vi "SCTL Sector Accumulation.vi"() -> (2 "Accummulated":T1(array[cluster]), 3 "New Data?":bool)   [LabVIEW 2013]
uses:
  Accumulated Count Array Fixed Point.ctl
  <vilib>/rvi/Memory/Memory_Emulation/niFpgaMemoryEmulationReadFromVariant.vi
  <vilib>/rvi/Emulation/niFpgaSctlEmulationGetInTimedLoop.vi
  <vilib>/rvi/Memory/Memory_Emulation/niFpgaMemoryEmulationWriteToVariant.vi
  <vilib>/rvi/DataTransferAndStorage/Container/Common/niFpgaContainerGetUniqueNameForEmu.vi
  <vilib>/rvi/FIFO/Fifo_Resource/nirvififoEmulationSetSize.vi
  <vilib>/rvi/Emulation/niFpgaSctlEmulationFifoFullMgr.vi
  <vilib>/rvi/errors/niFpgaSetErrorForExecOnDevCompSimple.vi
  <vilib>/rvi/eio/common/nirviEmuReportErrorAndStop.vi
  <vilib>/rvi/Emulation/niFpgaSctlEmulationResourceMgr.vi
  <vilib>/rvi/Memory/Memory_Emulation/nirvimemoryFastEmulation.vi
  <vilib>/rvi/Memory/Memory_Emulation/nirvimemoryEmulation.vi
  <vilib>/rvi/DataTransferAndStorage/Container/XNode/niFpgaContainer.xnode
  <vilib>/rvi/FIFO/Fifo_Resource/nirvififoEmulationRead.vi
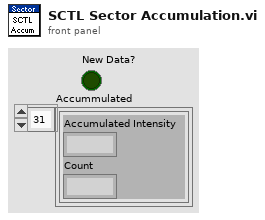
[diagram p1: front panel]
types:
  T1 = cluster{"Accumulated Intensity":fxp<+,20,20>, "Count":fxp<+,12,12>}[]
  T2 = cluster{"Accumulated Intensity":fxp<+,8,8>, "Count":fxp<+,1,1>}
  T3 = typedef "Accumulated Count Array Fixed Point.ctl" = cluster{"Accumulated Intensity":fxp<+,20,20>, "Count":fxp<+,12,12>}[]
  T4 = cluster{"Accumulated Intensity":fxp<+,21,21>, "Count":fxp<+,13,13>}[]
  T5 = cluster{"Accumulated Intensity":fxp<+,22,22>, "Count":fxp<+,14,14>}[]
  T6 = cluster{"Accumulated Intensity":fxp<+,23,23>, "Count":fxp<+,15,15>}[]
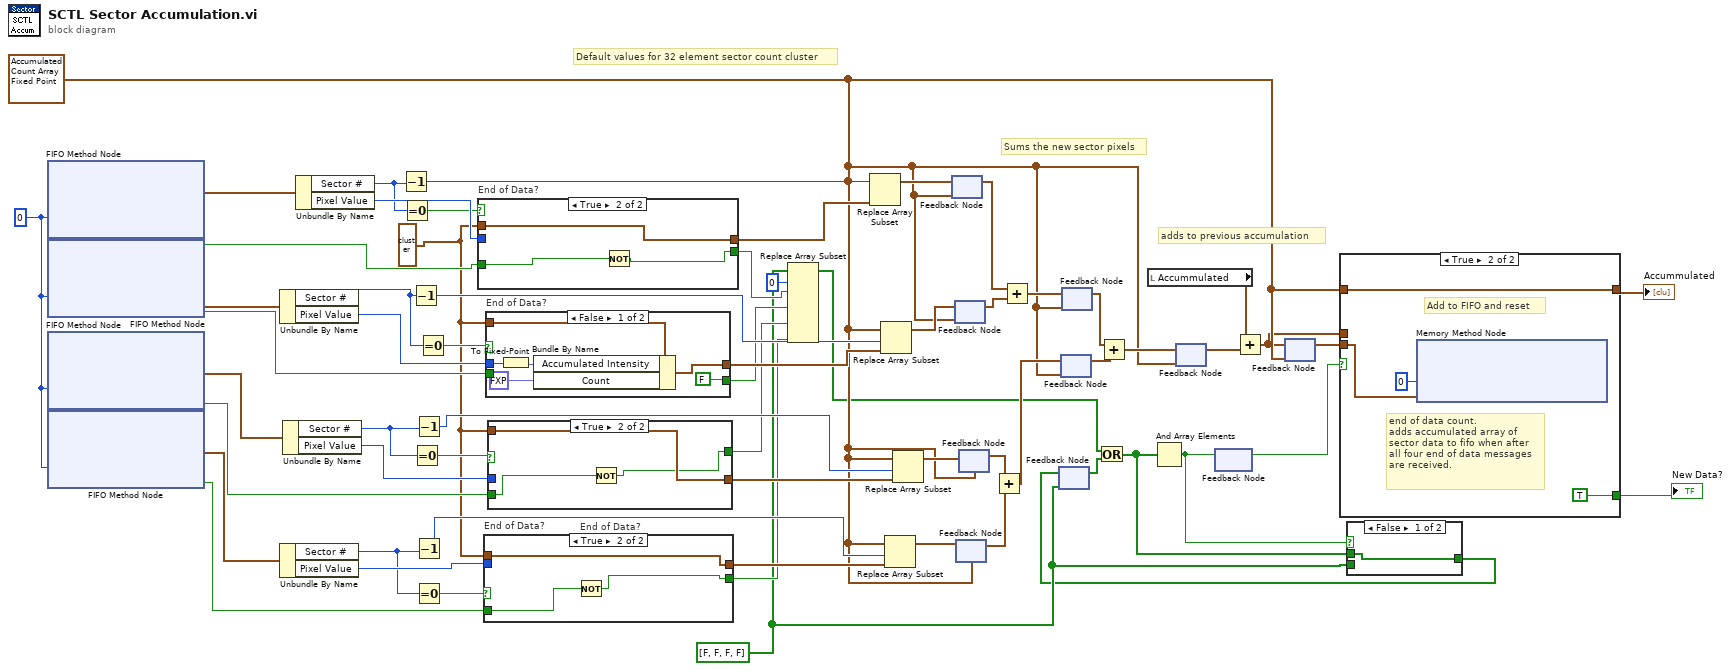
[diagram p0: block diagram]
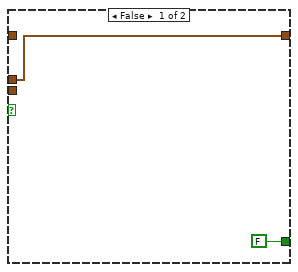
[diagram p3: hidden frame]
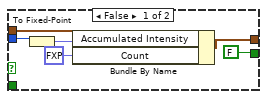
[diagram p4: hidden frame]
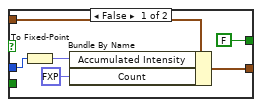
[diagram p5: hidden frame]
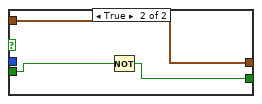
[diagram p6: hidden frame]
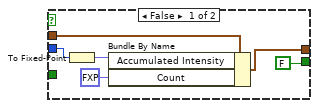
[diagram p7: hidden frame]
diagram:
  w2 = bool[] [FALSE, FALSE, FALSE, FALSE]
  w32 = T2 {"Accumulated Intensity"=0.0, "Count"=0.0} ("Accumulated Sector Cluster")
  w14 = T3 [{"Accumulated Intensity"=0.0, "Count"=0.0}, {"Accumulated Intensity"=0.0, "Count"=0.0}, {"Accumulated Intensity"=0.0, "Count"=0.0}, {"Accumulated Intensity"=0.0, "Count"=0.0}, {"Accumulated Intensity"=0.0, "Count"=0.0}, {"Accumulated Intensity"=0.0, "Count"=0.0}, {"Accumulated Intensity"=0.0, "Count"=0.0}, {"Accumulated Intensity"=0.0, "Count"=0.0}, {"Accumulated Intensity"=0.0, "Count"=0.0}, {"Accumulated Intensity"=0.0, "Count"=0.0}, {"Accumulated Intensity"=0.0, "Count"=0.0}, {"Accumulated Intensity"=0.0, "Count"=0.0}, {"Accumulated Intensity"=0.0, "Count"=0.0}, {"Accumulated Intensity"=0.0, "Count"=0.0}, {"Accumulated Intensity"=0.0, "Count"=0.0}, {"Accumulated Intensity"=0.0, "Count"=0.0}, {"Accumulated Intensity"=0.0, "Count"=0.0}, {"Accumulated Intensity"=0.0, "Count"=0.0}, {"Accumulated Intensity"=0.0, "Count"=0.0}, {"Accumulated Intensity"=0.0, "Count"=0.0}, {"Accumulated Intensity"=0.0, "Count"=0.0}, {"Accumulated Intensity"=0.0, "Count"=0.0}, {"Accumulated Intensity"=0.0, "Count"=0.0}, {"Accumulated Intensity"=0.0, "Count"=0.0}, {"Accumulated Intensity"=0.0, "Count"=0.0}, {"Accumulated Intensity"=0.0, "Count"=0.0}, {"Accumulated Intensity"=0.0, "Count"=0.0}, {"Accumulated Intensity"=0.0, "Count"=0.0}, {"Accumulated Intensity"=0.0, "Count"=0.0}, {"Accumulated Intensity"=0.0, "Count"=0.0}, {"Accumulated Intensity"=0.0, "Count"=0.0}, {"Accumulated Intensity"=0.0, "Count"=0.0}] ("Test Accumulated Array")
  w62 = 0 ("Timeout")
  # "adds to previous accumulation"
  # "Sums the new sector pixels"
  # "Default values for 32 element sector count cluster"
  n1 = xnode ("FIFO Method Node")("Timeout"=w62) -> ("Element"=w40:cluster{"Sector #":u8, "Pixel Value":u8}, "Timed Out?"=w36:bool)  [unwired: 1 in, 1 out]
  n2 = xnode ("FIFO Method Node")("Timeout"=w62) -> ("Element"=w39:cluster{"Sector #":u8, "Pixel Value":u8}, "Timed Out?"=w35:bool)  [unwired: 1 in, 1 out]
  n3 = xnode ("FIFO Method Node")("Timeout"=w62) -> ("Element"=w38:cluster{"Sector #":u8, "Pixel Value":u8}, "Timed Out?"=w34:bool)  [unwired: 1 in, 1 out]
  n4 = xnode ("FIFO Method Node")("Timeout"=w62) -> ("Element"=w37:cluster{"Sector #":u8, "Pixel Value":u8}, "Timed Out?"=w33:bool)  [unwired: 1 in, 1 out]
  n5 = Unbundle By Name(w39) -> ("Sector #"=w48:u8, "Pixel Value"=w58:u8)
  n6 = Unbundle By Name(w37) -> ("Sector #"=w44:u8, "Pixel Value"=w52:u8)
  n7 = Unbundle By Name(w38) -> ("Sector #"=w46:u8, "Pixel Value"=w55:u8)
  n8 = Unbundle By Name(w40) -> ("Sector #"=w50:u8, "Pixel Value"=w60:u8)
  n9 = Decrement(x=w50) -> (x-1=w61:u8)
  n10 = Equal To 0?(x=w50) -> (x = 0?=w49:bool)
  n11 = Decrement(x=w48) -> (x-1=w57:u8)
  n12 = Equal To 0?(x=w46) -> (x = 0?=w45:bool)
  n13 = Decrement(x=w46) -> (x-1=w41:u8)
  n14 = Decrement(x=w44) -> (x-1=w54:u8)
  n15 = Equal To 0?(x=w44) -> (x = 0?=w43:bool)
  n16 = Equal To 0?(x=w48) -> (x = 0?=w47:bool)
  n17 = case "End of Data?" shown="True" w49 {
    tunnel: w60 -> [w65 _]
    tunnel: [w68 w71] -> w59
    tunnel: w32 -> [w67 w71]
    tunnel: [FALSE w69] -> w10
    tunnel: w36 -> [_ w70]
    frame False {
      n18 = To Fixed-Point(number=w65) -> (fixed-point=w64:fxp<+,8,8>)  [unwired: 1 in]
      n19 = Bundle By Name(cluster=w67, "Accumulated Intensity"=w64, "Count"=fxp<+,1,1> 1.0) -> (w68:T2)
    }
    frame True {
      n20 = Not(x=w70) -> (.not. x?=w69:bool)
    }
  }
  n21 = case "End of Data?" shown="True" w43 {
    tunnel: [w77 w80] -> w53
    tunnel: w32 -> [w76 w80]
    tunnel: w52 -> [w73 _]
    tunnel: [FALSE w78] -> w7
    tunnel: w33 -> [_ w79]
    frame False {
      n22 = To Fixed-Point(number=w73) -> (fixed-point=w74:fxp<+,8,8>)  [unwired: 1 in]
      n23 = Bundle By Name(cluster=w76, "Accumulated Intensity"=w74, "Count"=fxp<+,1,1> 1.0) -> (w77:T2)
    }
    frame True {
      n24 = Not(x=w79) -> (.not. x?=w78:bool)
    }
  }
  n25 = case "End of Data?" shown="False" w47 {
    tunnel: w58 -> [w83 _]
    tunnel: w32 -> [w86 w89]
    tunnel: [w85 w89] -> w51
    tunnel: [FALSE w87] -> w9
    tunnel: w35 -> [_ w88]
    frame False {
      n26 = To Fixed-Point(number=w83) -> (fixed-point=w82:fxp<+,8,8>)  [unwired: 1 in]
      n27 = Bundle By Name(cluster=w86, "Accumulated Intensity"=w82, "Count"=fxp<+,1,1> 1.0) -> (w85:T2)
    }
    frame True {
      n28 = Not(x=w88) -> (.not. x?=w87:bool)
    }
  }
  n29 = case "End of Data?" shown="True" w45 {
    tunnel: [w95 w98] -> w56
    tunnel: w55 -> [w92 _]
    tunnel: w32 -> [w94 w98]
    tunnel: [FALSE w96] -> w8
    tunnel: w34 -> [_ w97]
    frame False {
      n30 = To Fixed-Point(number=w92) -> (fixed-point=w91:fxp<+,8,8>)  [unwired: 1 in]
      n31 = Bundle By Name(cluster=w94, "Accumulated Intensity"=w91, "Count"=fxp<+,1,1> 1.0) -> (w95:T2)
    }
    frame True {
      n32 = Not(x=w97) -> (.not. x?=w96:bool)
    }
  }
  n33 = Replace Array Subset(array=w2, new element #1=w10, index #1=0 ("index"), new element #2=w9, new element #3=w8, new element #4=w7) -> (w6:bool[])  [unwired: 3 in]
  n34 = Replace Array Subset(array=w14, new element=w59, index=w61) -> (w29:T3)
  n35 = Replace Array Subset(array=w14, new element=w51, index=w57) -> (w27:T3)
  n36 = Replace Array Subset(array=w14, new element=w53, index=w54) -> (w23:T3)
  n37 = Replace Array Subset(array=w14, new element=w56, index=w41) -> (w25:T3)
  n38 = feedback #1(w14) -> (w28:T3)
  n39 = feedback-in #1(w29) -> ()
  n40 = feedback #2(w14) -> (w26:T3)
  n41 = feedback-in #2(w27) -> ()
  n42 = feedback #3(w14) -> (w22:T3)
  n43 = feedback-in #3(w23) -> ()
  n44 = feedback #4(w14) -> (w24:T3)
  n45 = feedback-in #4(w25) -> ()
  n46 = Add(x=w24, y=w22) -> (x+y=w19:T4)
  n47 = Add(x=w28, y=w26) -> (x+y=w21:T4)
  n48 = feedback #5(w2) -> (w12:bool[])
  n49 = feedback #6(w14) -> (w18:T4)
  n50 = feedback-in #6(w19) -> ()
  n51 = feedback #7(w14) -> (w20:T4)
  n52 = feedback-in #7(w21) -> ()
  n53 = Or(x=w6, y=w12) -> (x .or. y?=w3:bool[])
  n54 = Add(x=w20, y=w18) -> (x+y=w17:T5)
  n55 = local read "Accummulated"() -> (w31:T1)
  n56 = And Array Elements(Boolean array=w3) -> (logical AND=w4:bool)
  n57 = feedback #8(w14) -> (w16:T5)
  n58 = feedback-in #8(w17) -> ()
  n59 = feedback #9() -> (w5:bool)  [unwired: 1 in]
  n60 = feedback-in #9(w4) -> ()
  n61 = Add(x=w31, y=w16) -> (x+y=w13:T6)
  n62 = feedback #10(w14) -> (w15:T6)
  n63 = feedback-in #10(w13) -> ()
  n64 = case shown="True" w5 {
    tunnel: w15 -> [_ w101]
    tunnel: w14 -> [_ w102]
    tunnel: [FALSE ("New Data?") TRUE ("New Data?")] -> w42
    tunnel: [w99 w102] -> w30
    tunnel: w13 -> [w99 _]
    frame False {
    }
    frame True {
      # "end of data count.\nadds accumulated array of\nsector data to fifo when after\nall four end of data messages\nare received."
      # "Add to FIFO and reset"
      n65 = xnode ("Memory Method Node")("Address"=u32 0, "Data"=w101) -> ()  [unwired: 1 in, 1 out]
    }
  }
  "New Data?" <- w42
  "Accummulated" <- w30
  n66 = case shown="False" w4 {
    tunnel: w3 -> [w105 _]
    tunnel: w2 -> [_ w106]
    tunnel: [w105 w106] -> w1
    frame False {
    }
    frame True {
    }
  }
  n67 = feedback-in #5(w1) -> ()
